vi "getFromDisplay.vi"(8 "error in (no error)":errorcluster, 11 "PixelflySettings in":refnum<class "PixelflySettings.lvclass">) -> (0 "error out":errorcluster, 3 "PixelflySettings out":refnum<class "PixelflySettings.lvclass">)   [LabVIEW 2009, in "Tools.lvlib" / "Settings.lvlib" / "PixelflySettings.lvclass"]
uses:
  PixelflySettings.lvclass
  PixelflySettings.lvclass/PixelflySettings.ctl
  CamaraSettings.lvclass
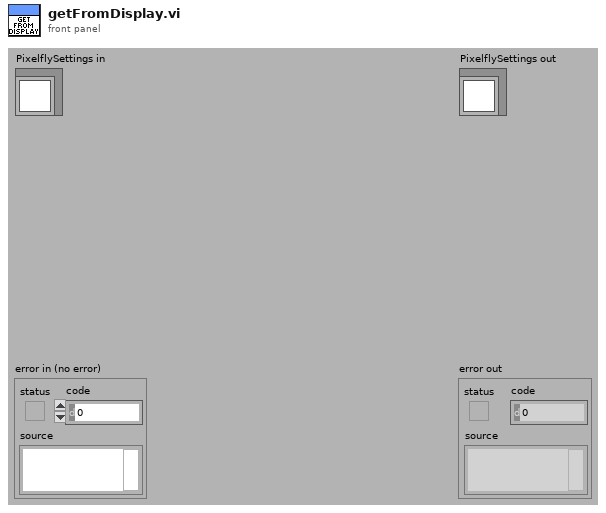
[diagram p1: front panel]
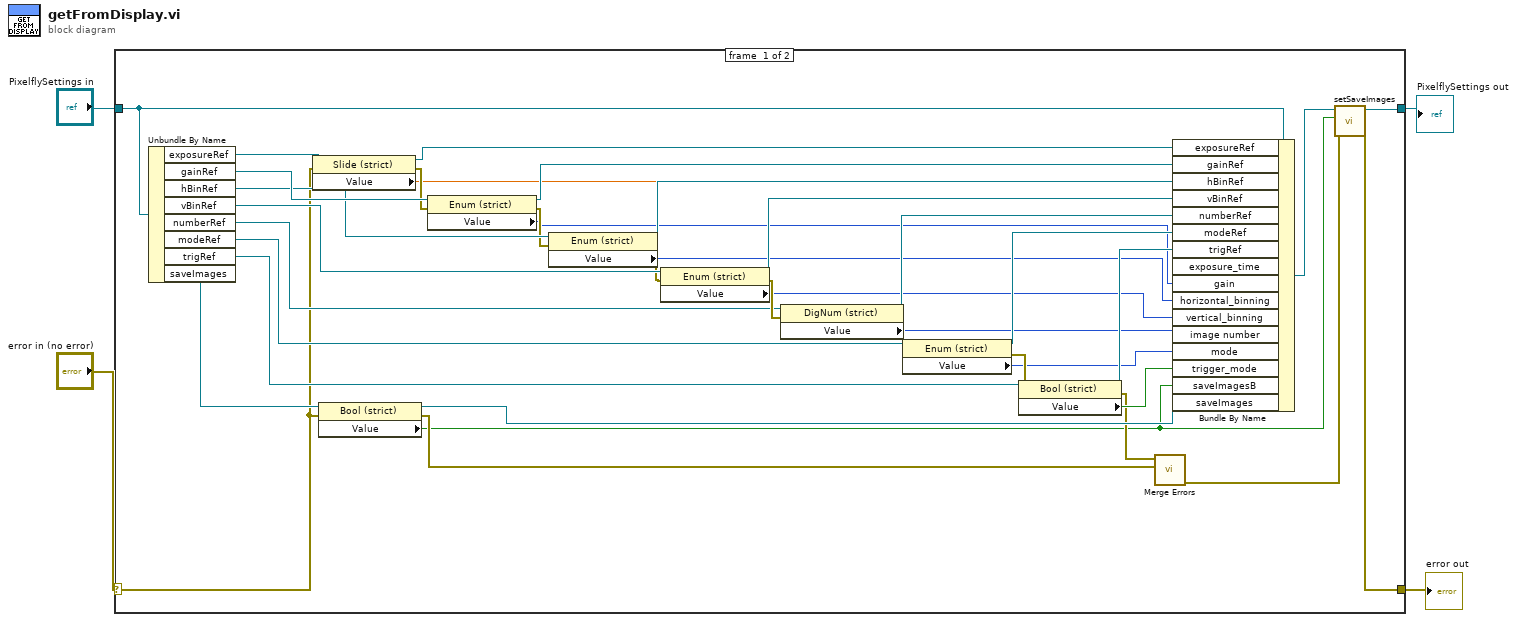
[diagram p0: block diagram]
diagram:
  n1 = case shown="No Error" "error in (no error)" {
    selector: "error in (no error)" -> [w13 w44]
    tunnel: [w6 w44] -> w1
    tunnel: [w5 w43] -> w2
    tunnel: "PixelflySettings in" -> [w22 w43]
    frame #0 {
      n2 = Unbundle By Name(w22) -> ("exposureRef"=w42:refnum<vi>, "gainRef"=w41:refnum<vi>, "hBinRef"=w39:refnum<vi>, "vBinRef"=w37:refnum<vi>, "numberRef"=w34:refnum<vi>, "modeRef"=w33:refnum<vi>, "trigRef"=w31:refnum<vi>, "saveImages"=w14:refnum<vi>)
      n3 = property class="Slide (strict)"(reference=w42, error in=w13) -> (reference out=w29:refnum<vi>, error out=w40:errorcluster, "Value"=w21:dbl)
      n4 = property class="Bool (strict)"(reference=w14, error in=w13) -> (reference out=w12:refnum<vi>, error out=w11:errorcluster, "Value"=w8:bool)
      n5 = property class="Enum (strict)"(reference=w41, error in=w40) -> (reference out=w28:refnum<vi>, error out=w38:errorcluster, "Value"=w20:enum16{"Low", "High"})
      n6 = property class="Enum (strict)"(reference=w39, error in=w38) -> (reference out=w27:refnum<vi>, error out=w36:errorcluster, "Value"=w19:enum16{"1", "2"})
      n7 = property class="Enum (strict)"(reference=w37, error in=w36) -> (reference out=w26:refnum<vi>, error out=w35:errorcluster, "Value"=w18:enum16{"1", "2"})
      n8 = property class="DigNum (strict)"(reference=w34, error in=w35) -> (reference out=w25:refnum<vi>, error out=w32:errorcluster, "Value"=w17:i32)
      n9 = property class="Enum (strict)"(reference=w33, error in=w32) -> (reference out=w24:refnum<vi>, error out=w30:errorcluster, "Value"=w16:enum16{"Asynch Shutter", "Double Shot", "Video"})
      n10 = property class="Bool (strict)"(reference=w31, error in=w30) -> (reference out=w23:refnum<vi>, error out=w10:errorcluster, "Value"=w15:bool)
      n11 = call <vilib>:"Merge Errors.vi"("error in 2 (no error)"=w11, "error in 1 (no error)"=w10) -> ("error out"=w7:errorcluster)  [unwired: 5 in]
      n12 = Bundle By Name(cluster=w22, "exposureRef"=w29, "gainRef"=w28, "hBinRef"=w27, "vBinRef"=w26, "numberRef"=w25, "modeRef"=w24, "trigRef"=w23, "exposure_time"=w21, "gain"=w20, "horizontal_binning"=w19, "vertical_binning"=w18, "image number"=w17, "mode"=w16, "trigger_mode"=w15, "saveImagesB"=w8, "saveImages"=w12) -> (w9:refnum<class "PixelflySettings.lvclass">)
      n13 = call "setSaveImages.vi"("error in (no error)"=w7, "saveImages"=w8, "CamaraSettings in"=w9) -> ("error out"=w6:errorcluster, "CamaraSettings out"=w5:refnum<class "PixelflySettings.lvclass">)  [unwired: 7 in]
    }
    frame #1 {
    }
  }
  "error out" <- w1
  "PixelflySettings out" <- w2
